vi "test massdataInlvlibp.vi"() -> ()   [LabVIEW 2017]
uses:
  addons/MassData-Parameter/Utility/Def-MassData Status Indicator(Vertical).ctl
  8bf0d7f0-6af5-4b65-a942-963b60026253.vi
  addons/MassData-Parameter/_support/FGV-MassData(lvlibp).vi
  massdataInlvlibp.lvlib
panel:
  in  "MassData Status":T1 {"r" scale=1.0..1000000.0 scale format="%#_6p"; "w" scale=1.0..1000000.0 scale format="%#_6p"}
  in  "stop":bool
  out "unpacked source data 1":waveform(dbl)(graph)
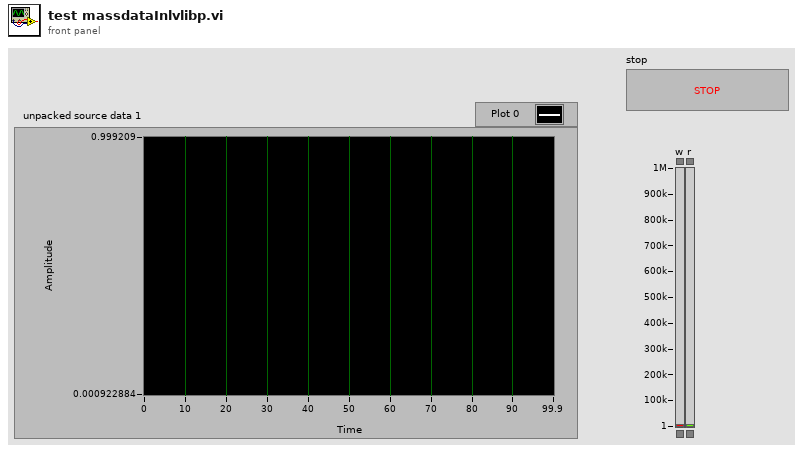
[diagram p1: front panel]
types:
  T1 = typedef "Def-MassData Status Indicator(Vertical).ctl" = cluster{"w":cluster{dbl, dbl}, "r":cluster{dbl, dbl}}
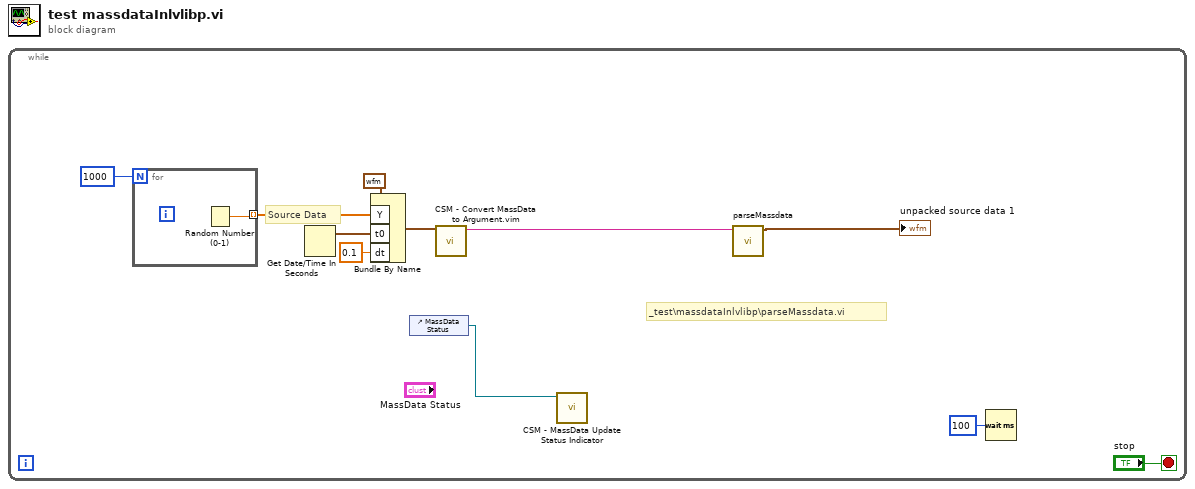
[diagram p0: block diagram]
diagram:
  n1 = while {
    stop <- "stop" stop-if-true
    # "_test\\massdataInlvlibp\\parseMassdata.vi"
    # "Source Data"
    n2 = for {
      N: 1000 -> [_]
      tunnel: [w12] -> w7 mode=indexing
      n3 = Random Number (0-1)() -> (number: 0 to 1=w12:dbl)
    }
    n4 = Get Date/Time In Seconds() -> (seconds since 1Jan1904=w9:timestamp)
    n5 = Bundle By Name(cluster=waveform(dbl) {"t0"=timestamp(0 s since 1904-01-01), "dt"=1.0, "Y"=[]} ("Waveform"), "Y"=w7, "t0"=w9, "dt"=0.1) -> (w6:waveform(dbl))
    n6 = control-ref of="MassData Status"() -> (w1:refnum<vi>)
    n7 = call "CSM - Convert MassData to Argument.vim"("DBL"=w6) -> ("MassData Argument"=w5:string)  [unwired: 7 in, 1 out]
    n8 = call "CSM - MassData Update Status Indicator.vi"("MassData Status Indicator"=w1) -> ()  [unwired: 10 in, 1 out]
    n9 = call "parseMassdata.vi"("Arguments"=w5) -> ("unpacked source data 1"=→"unpacked source data 1":waveform(dbl))  [unwired: 10 in]
    n10 = Wait (ms)(milliseconds to wait=u32 100) -> ()  [unwired: 1 out]
  }
